vi "Double and Triple Letter Box IDs.vi"(8 "Error In":errorcluster, 11 "1D String Array":string[](array[string])=["abcdef", "bababc", "abbcde", "abcccd", "aabcdd", "abcdee", "ababab"]) -> (0 "Error Out":errorcluster, 2 "Triples":i32, 3 "Doubles":i32)   [LabVIEW 2019]
doc: "Given a 1D String array, determine how many of the strings have characters that repeat -exactly- 2 times, and -exactly- 3 times. If a string has two repeats of the same kind (e.g. 2 characters repeat 2 times) it only counts once."
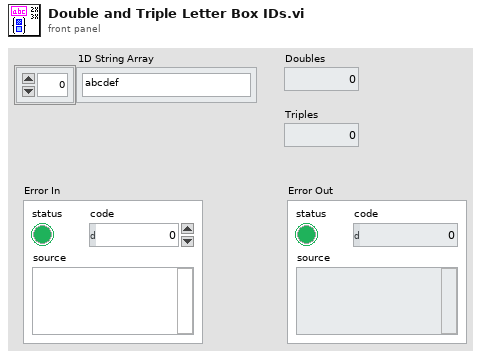
[diagram p1: front panel]
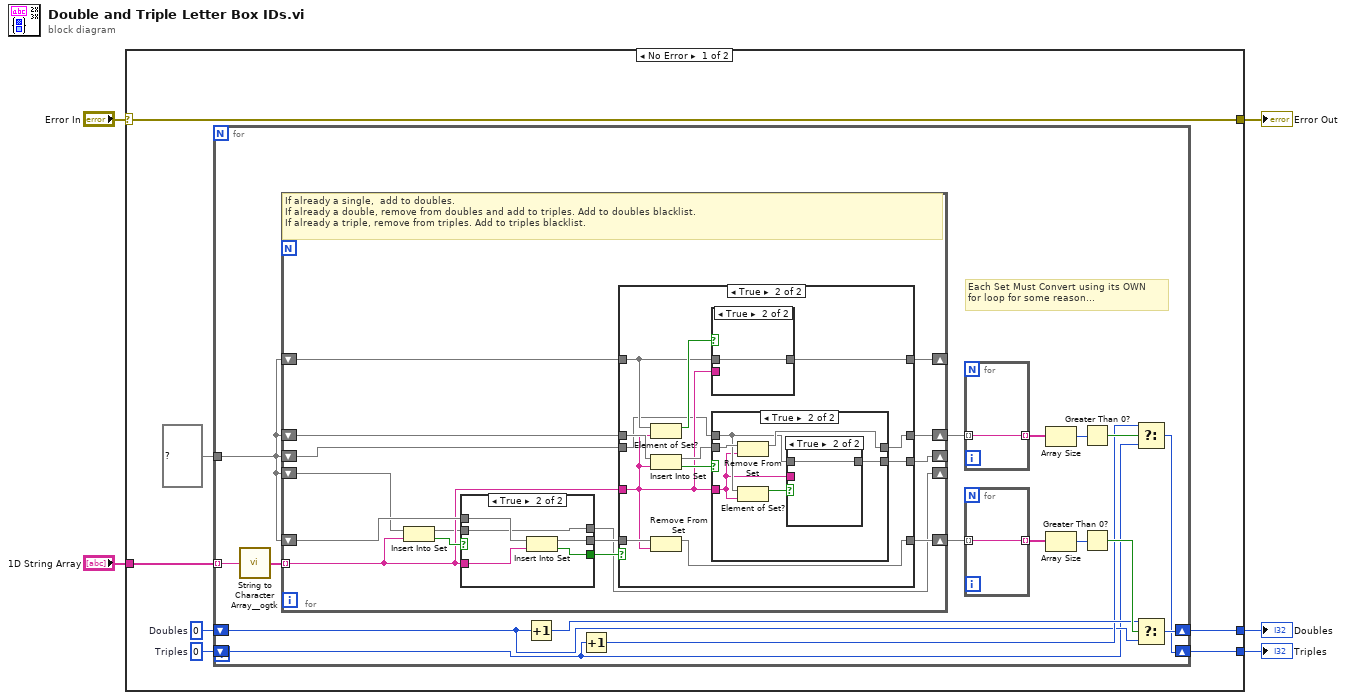
[diagram p0: block diagram]
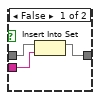
[diagram p4: hidden frame]
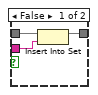
[diagram p6: hidden frame]
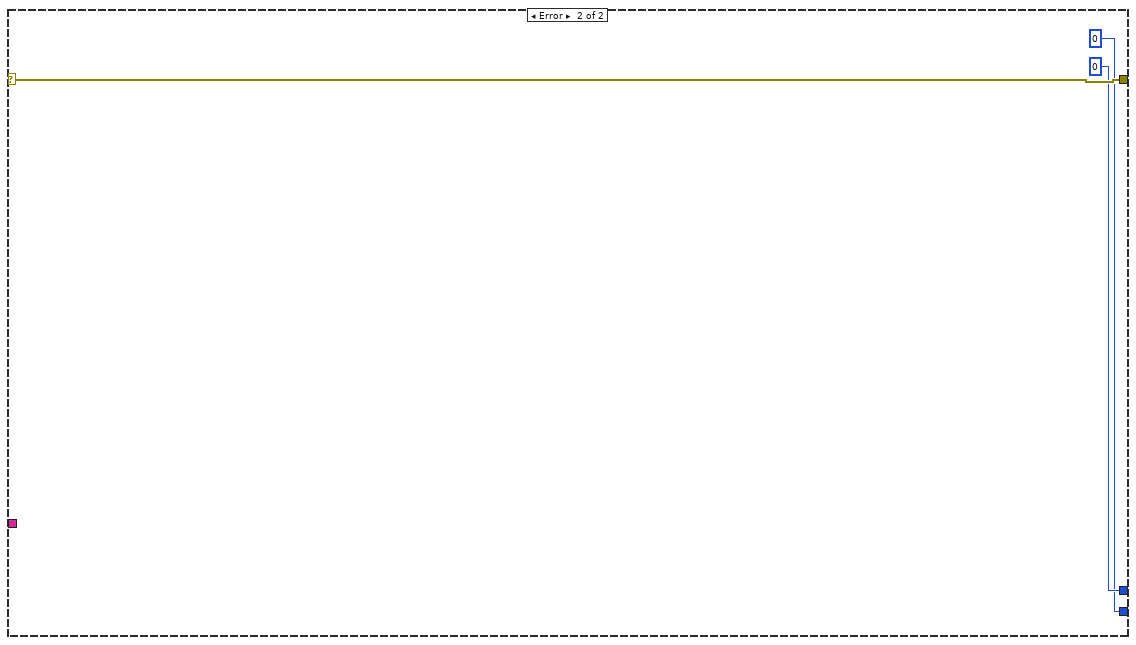
[diagram p7: hidden frame]
diagram:
  n1 = case shown="No Error" "Error In" {
    selector: "Error In" -> [w6 w89]
    tunnel: [w12 0 ("Triples")] -> w5
    tunnel: [w11 0 ("Doubles")] -> w4
    tunnel: "1D String Array" -> [w8 _]
    tunnel: [w6 w89] -> w1
    frame No Error {
      w10 = 0  # Triples
      w9 = 0  # Doubles
      n2 = for {
        tunnel: w8 -> [w29] mode=indexing
        shift-right: [w18] -> w11
        shift-left: w9 -> [w19]
        shift-right: [w16] -> w12
        shift-left: w10 -> [w17]
        tunnel: set{string} {} ("set in") -> [w13]
        # "Each Set Must Convert using its OWN\nfor loop for some reason..."
        n3 = call <userlib>:"String to Character Array__ogtk.vi"("Input String"=w29) -> ("Character Array"=w28:string[])
        n4 = for {
          tunnel: w28 -> [w38] mode=indexing
          shift-right: [w42] -> w15
          shift-left: w13 -> [w46]
          shift-right: [w41] -> w27
          shift-left: w13 -> [w43]
          shift-right: [w36] -> _
          shift-left: w13 -> [w40]
          shift-right: [w34] -> _
          shift-left: w13 -> [w35]
          shift-right: [w32] -> _
          shift-left: w13 -> [w33]
          # "If already a single,  add to doubles. \nIf already a double, remove from doubles and add to triples. Add to doubles blacklist. \nIf already a triple, remove from triples. Add to triples blacklist."
          n5 = Insert Into Set(10:w38, 11:w40) -> (2:w39:bool, 3:w37:set{string})
          n6 = case shown="True" w39 {
            selector: w39 -> [w49 _]
            tunnel: w46 -> [w48 w54]
            tunnel: [w49 w53] -> w45
            tunnel: [w48 w52] -> w44
            tunnel: w38 -> [_ w51]
            tunnel: w37 -> [w47 w50]
            tunnel: [w47 w50] -> w36
            frame False {
            }
            frame True {
              n7 = Insert Into Set(10:w51, 11:w54) -> (2:w53:bool, 3:w52:set{string})
            }
          }
          n8 = case shown="True" w45 {
            tunnel: w44 -> [w58 w70]
            tunnel: w38 -> [_ w62]
            tunnel: w43 -> [w57 w69]
            tunnel: [w58 w66] -> w42
            tunnel: [w57 w65] -> w41
            tunnel: w35 -> [w56 w63]
            tunnel: [w56 w61] -> w34
            tunnel: w33 -> [w55 w60]
            tunnel: [w55 w59] -> w32
            frame False {
            }
            frame True {
              n9 = Element of Set?(10:w62, 11:w63) -> (3:w64:bool)
              n10 = Insert Into Set(10:w62, 11:w69) -> (2:w68:bool, 3:w67:set{string})
              n11 = Remove From Set(10:w62, 11:w70) -> (3:w66:set{string})  [unwired: 1 out]
              n12 = case shown="True" w64 {
                tunnel: w63 -> [w73 w74]
                tunnel: w62 -> [w72 _]
                tunnel: [w71 w74] -> w61
                frame False {
                  n13 = Insert Into Set(10:w72, 11:w73) -> (3:w71:set{string})  [unwired: 1 out]
                }
                frame True {
                }
              }
              n14 = case shown="True" w68 {
                tunnel: w62 -> [_ w78]
                tunnel: w67 -> [w76 w82]
                tunnel: [w76 w81] -> w65
                tunnel: w60 -> [w75 w79]
                tunnel: [w75 w77] -> w59
                frame False {
                }
                frame True {
                  n15 = Remove From Set(10:w78, 11:w82) -> (3:w81:set{string})  [unwired: 1 out]
                  n16 = Element of Set?(10:w78, 11:w79) -> (3:w80:bool)
                  n17 = case shown="True" w80 {
                    tunnel: w79 -> [w85 w86]
                    tunnel: w78 -> [w84 _]
                    tunnel: [w83 w86] -> w77
                    frame False {
                      n18 = Insert Into Set(10:w84, 11:w85) -> (3:w83:set{string})  [unwired: 1 out]
                    }
                    frame True {
                    }
                  }
                }
              }
            }
          }
        }
        n19 = Increment(x=w19) -> (x+1=w21:i32)
        n20 = Increment(x=w17) -> (x+1=w20:i32)
        n21 = for {
          tunnel: w27 -> [w31] mode=indexing
          tunnel: [w31] -> w26 mode=indexing
        }
        n22 = for {
          tunnel: [w30] -> w14 mode=indexing
          tunnel: w15 -> [w30] mode=indexing
        }
        n23 = Array Size(array=w26) -> (size(s)=w24:i32)
        n24 = Array Size(array=w14) -> (size(s)=w25:i32)
        n25 = Greater Than 0?(x=w24) -> (x > 0?=w22:bool)
        n26 = Greater Than 0?(x=w25) -> (x > 0?=w23:bool)
        n27 = Select(t=w20, s=w22, f=w17) -> (s? t:f=w16:i32)
        n28 = Select(t=w21, s=w23, f=w19) -> (s? t:f=w18:i32)
      }
    }
    frame Error {
    }
  }
  "Triples" <- w5
  "Doubles" <- w4
  "Error Out" <- w1
